vi "Phasor_Abort Parallel Computation.vi"() -> ()   [LabVIEW 2019]
panel:
  out "Abort Parallel Computation":bool
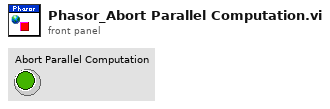
[diagram p1: front panel]
diagram:
